vi "Buffer Initialize.vi"(8 "error in (no error)":errorcluster, 9 "Number Of Elements":i32, 10 "Sector Number":i32, 11 "1D U16 Group With ID DVR Queue in":refnum<class "1D U16 Group With ID DVR Queue.lvclass">) -> (0 "error out":errorcluster, 3 "1D U16 Group With ID DVR Queue out":refnum<class "1D U16 Group With ID DVR Queue.lvclass">)   [LabVIEW 2019, in "1D U16 Group With ID DVR Queue.lvclass"]
uses:
  1D U16 Group With ID DVR Queue.lvclass
  Type Def/Data Type.ctl
  1D U16 Group With ID DVR Queue.lvclass/1D U16 Group With ID DVR Queue.ctl
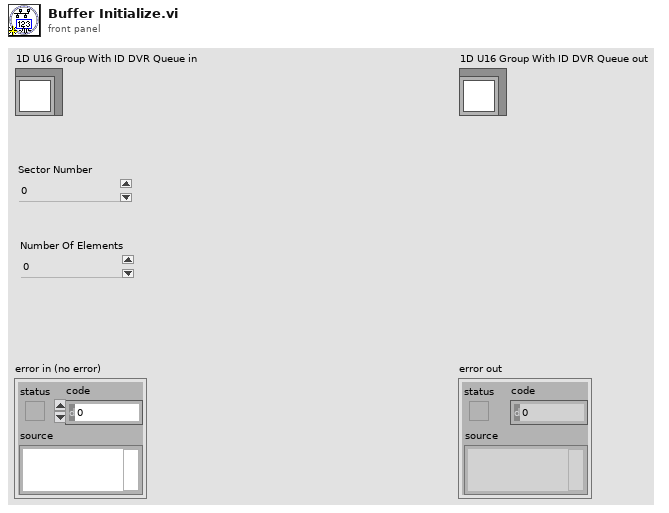
[diagram p1: front panel]
types:
  T1 = typedef "Data Type.ctl" = cluster{"Data ID":i64, "U16 Data Group":cluster{"Array":u16[]}[]}
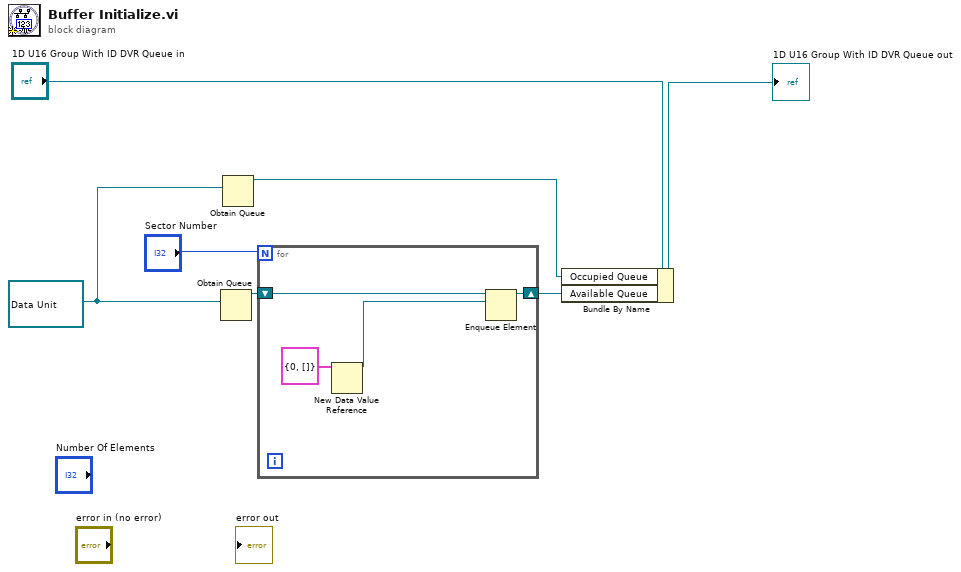
[diagram p0: block diagram]
diagram:
  w4 = refnum<data-value> refnum ("data value reference")
  n1 = Obtain Queue(element data type=w4) -> (queue out=w7:refnum<queue>)  [unwired: 4 in, 2 out]
  n2 = Obtain Queue(element data type=w4) -> (queue out=w5:refnum<queue>)  [unwired: 4 in, 2 out]
  n3 = for {
    N: "Sector Number" -> [_]
    shift-right: [w10] -> w6
    shift-left: w7 -> [w11]
    n4 = New Data Value Reference(data value=T1 {"Data ID"=0, "U16 Data Group"=[]} ("Data Unit")) -> (data value reference=w8:refnum<data-value>)  [unwired: 1 in, 1 out]
    n5 = Enqueue Element(queue=w11, element=w8) -> (queue out=w10:refnum<queue>)  [unwired: 2 in, 2 out]
  }
  n6 = Bundle By Name(cluster="1D U16 Group With ID DVR Queue in", "Occupied Queue"=w5, "Available Queue"=w6) -> (→"1D U16 Group With ID DVR Queue out":refnum<class "1D U16 Group With ID DVR Queue.lvclass">)
